vi "Write FPGAVIRef.vi"(8 "error in (no error)":errorcluster, 10 "FPGAVIRef":refnum<k20>, 11 "FPGATarget in":refnum<class "FPGATarget.lvclass">) -> (0 "error out":errorcluster, 3 "FPGATarget out":refnum<class "FPGATarget.lvclass">)   [LabVIEW 2013, in "FPGATarget.lvclass"]
uses:
  FPGATarget.lvclass
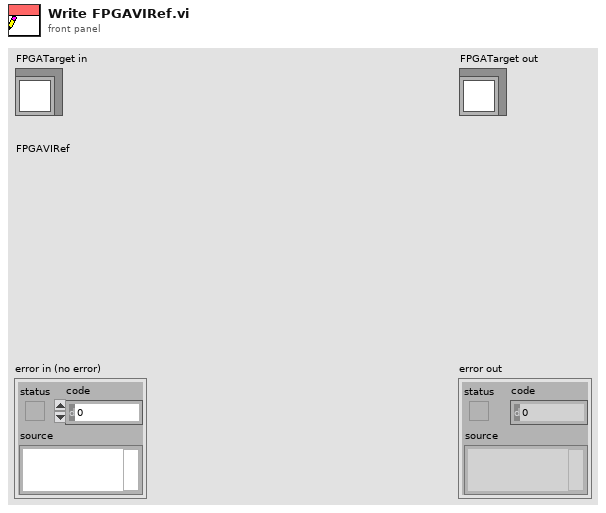
[diagram p1: front panel]
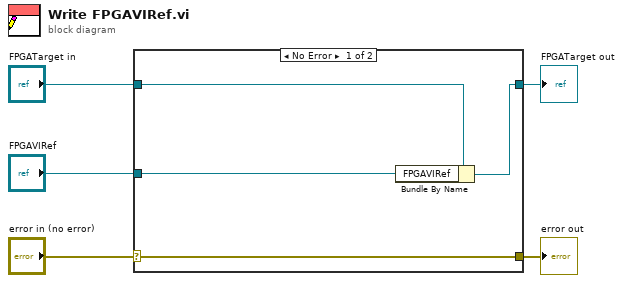
[diagram p0: block diagram]
diagram:
  n1 = case shown="No Error" "error in (no error)" {
    selector: "error in (no error)" -> [w9 w10]
    tunnel: [w9 w10] -> w4
    tunnel: [w7 w11] -> w2
    tunnel: "FPGATarget in" -> [w8 w11]
    tunnel: "FPGAVIRef" -> [w6 _]
    frame No Error {
      n2 = Bundle By Name(cluster=w8, "FPGAVIRef"=w6) -> (w7:refnum<class "FPGATarget.lvclass">)
    }
    frame Error {
    }
  }
  "error out" <- w4
  "FPGATarget out" <- w2
